vi "usb write reg length.vi"(11 "lengthToWrite":i32) -> (3 "function return":bool)   [LabVIEW 2018, in "Dll1_x64_191014_0.lvlib"]
doc: "__declspec(dllexport) bool usb_write_reg_length(int lengthToWrite);"
uses:
  Dll1_x64_191014_0.lvlib
  Dll1.dll
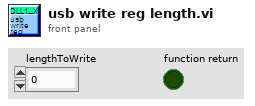
[diagram p1: front panel]
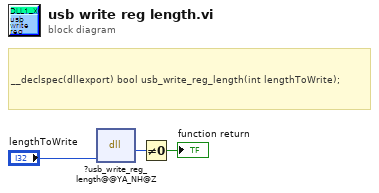
[diagram p0: block diagram]
diagram:
  # "__declspec(dllexport) bool usb_write_reg_length(int lengthToWrite);"
  n1 = dll-call lib="PTH2zabs CUsersLenovoDesktopDHCC실험2#lux image capture_0.9.1.1_Temporaryuser.libDll1_x64_191014_0Dll1.*" fn="?usb_write_reg_length@@YA_NH@Z"("lengthToWrite"="lengthToWrite") -> (w2:u8)  [unwired: 4 in, 2 out]
  n2 = Not Equal To 0?(x=w2) -> (x != 0?=→"function return":bool)
